vi "定点周期设置.vi"(11 "TimingControl 输入":refnum<class "TimingControl.lvclass">) -> (3 "TimingControl 输出":refnum<class "TimingControl.lvclass">)   [LabVIEW 2016, in "ZKTimingControl.lvlib" / "TimingControl.lvclass"]
uses:
  TimingControl.lvclass
  <vilib>/Utility/miscctls.llb/LVPointTypeDef.ctl
  TimingControl.lvclass/TimingControl.ctl
  <vilib>/Utility/miscctls.llb/LVPositionTypeDef.ctl
panel:
  out "时间标识":timestamp format="%<%x %X>T"
  in  "每月启动":T1
  in  "每周启动":T2
  out "测试状态.结束时间":timestamp caption="结束时间" format="%<%y/%m/%d %H:%M:%S>T"
  out "测试状态.启动次数":dbl caption="启动次数"
  out "测试状态.启动时间":timestamp caption="启动时间" format="%<%y/%m/%d %H:%M:%S>T"
  in  "测量参数":T3={"氨氮"=TRUE, "总磷"=TRUE, "总氮"=TRUE, "CODMn"=TRUE, "CODCr"=FALSE, "氟化物"=FALSE, "挥发酚"=FALSE}
  in  "保存":bool
  in  "退出":bool
  in  "批量设置":bool
  out "周期模式选择卡":enum32{"选项卡 1", "选项卡 2"}(tab)
  in  "定点周期":T4
  in  "间隔启动":T6
  in  "周期模式":T7
  # "分钟"
  # "次"
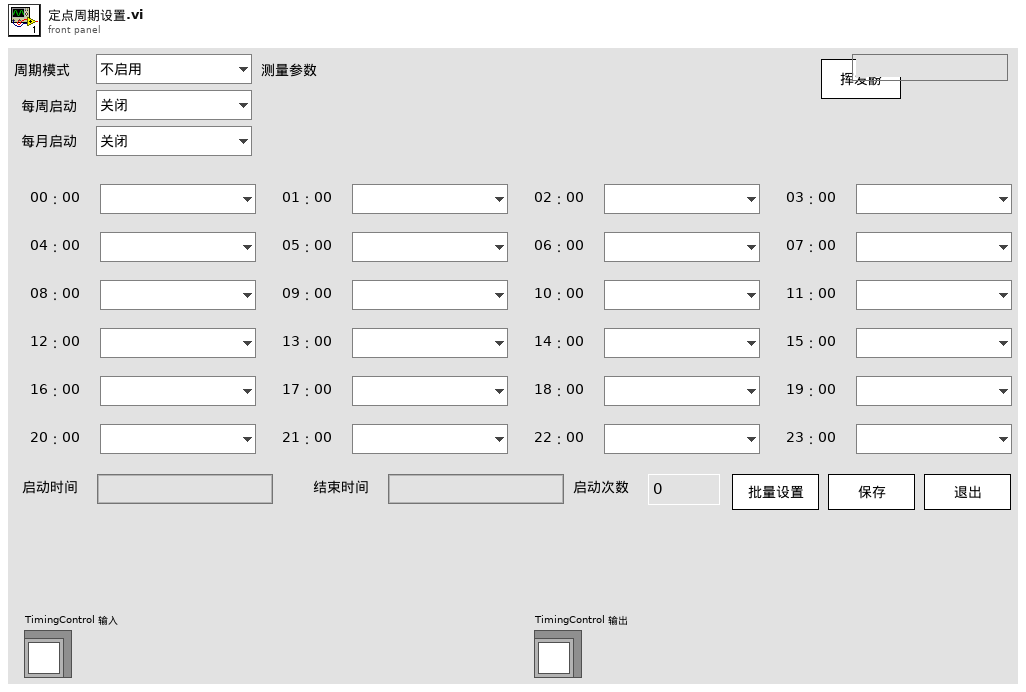
[diagram p1: front panel]
types:
  T1 = typedef "ZKTimingControl.lvlib/TimingControl.lvclass/每月启动.ctl" = enum16{"关闭", "1号", "2号", "3号", "4号", "5号", "6号", "7号", "8号", "9号", "10号", "11号", "12号", "13号", "14号", "15号", "16号", "17号", "18号", "19号", "20号", "21号", "22号", "23号", "24号", "25号", "26号", "27号", "28号", "29号", "30号", "31号"}
  T2 = typedef "ZKTimingControl.lvlib/TimingControl.lvclass/每周启动.ctl" = enum16{"关闭", "周日", "周一", "周二", "周三", "周四", "周五", "周六"}
  T3 = typedef "ZKTimingControl.lvlib/TimingControl.lvclass/测量参数.ctl" = cluster{"氨氮":bool, "总磷":bool, "总氮":bool, "CODMn":bool, "CODCr":bool, "氟化物":bool, "挥发酚":bool}
  T4 = typedef "ZKTimingControl.lvlib/TimingControl.lvclass/定点周期设置.ctl" = cluster{"启动命令":T5, "启动命令 2":T5, "启动命令 3":T5, "启动命令 4":T5, "启动命令 5":T5, "启动命令 6":T5, "启动命令 7":T5, "启动命令 8":T5, "启动命令 9":T5, "启动命令 10":T5, "启动命令 11":T5, "启动命令 12":T5, "启动命令 13":T5, "启动命令 14":T5, "启动命令 15":T5, "启动命令 16":T5, "启动命令 17":T5, "启动命令 18":T5, "启动命令 19":T5, "启动命令 20":T5, "启动命令 21":T5, "启动命令 22":T5, "启动命令 23":T5, "启动命令 24":T5}
  T5 = typedef "ZKTimingControl.lvlib/TimingControl.lvclass/启动命令选择.ctl" = enum16{"", "加标回收（启动采配水）", "加标回收（不启动采配水）", "水样测试（启动采配水）", "水样测试（不启动采配水）", "平行样测试（启动采配水）", "平行样测试（不启动采配水）", "集成干预测试"}
  T6 = typedef "ZKTimingControl.lvlib/TimingControl.lvclass/间隔启动设置.ctl" = cluster{"启动命令":T5, "启动间隔":dbl, "启动次数":i32}
  T7 = typedef "ZKTimingControl.lvlib/TimingControl.lvclass/周期模式设置.ctl" = enum16{"不启用", "定点模式", "间隔模式"}
  T8 = typedef "LVPointTypeDef.ctl" = cluster{"Horizontal":i16, "Vertical":i16}
  T9 = typedef "LVPositionTypeDef.ctl" = cluster{"Left":i32, "Top":i32}
  T10 = cluster{"启动时间":timestamp, "结束时间":timestamp, "启动次数":dbl}
  T11 = typedef "ZKTimingControl.lvlib/TimingControl.lvclass/State Data.ctl" = cluster{"仪器时间":timestamp, "仪器运行状态":bool, "配置文件路径":path, "测量参数":T3, "测试状态":cluster{"启动时间":timestamp, "结束时间":timestamp, "启动次数":dbl}, "配置信息":T12}
  T12 = typedef "ZKTimingControl.lvlib/TimingControl.lvclass/配置信息.ctl" = cluster{"每周启动":T2, "每月启动":T1, "周期模式":T7, "测量参数":T3, "定点周期":T4, "间隔启动":T6, "配置时间":timestamp}
  T13 = typedef "周期设置.lvlib/周期模式设置.ctl" = enum16{"不启用", "定点模式", "间隔模式"}
  T14 = cluster{"每周启动":T2, "每月启动":T1, "周期模式":T7, "测量参数":T3, "定点周期":T4, cluster{"启动命令":T5, "启动间隔":dbl, "启动次数":i32}, "seconds since 1Jan1904":timestamp}
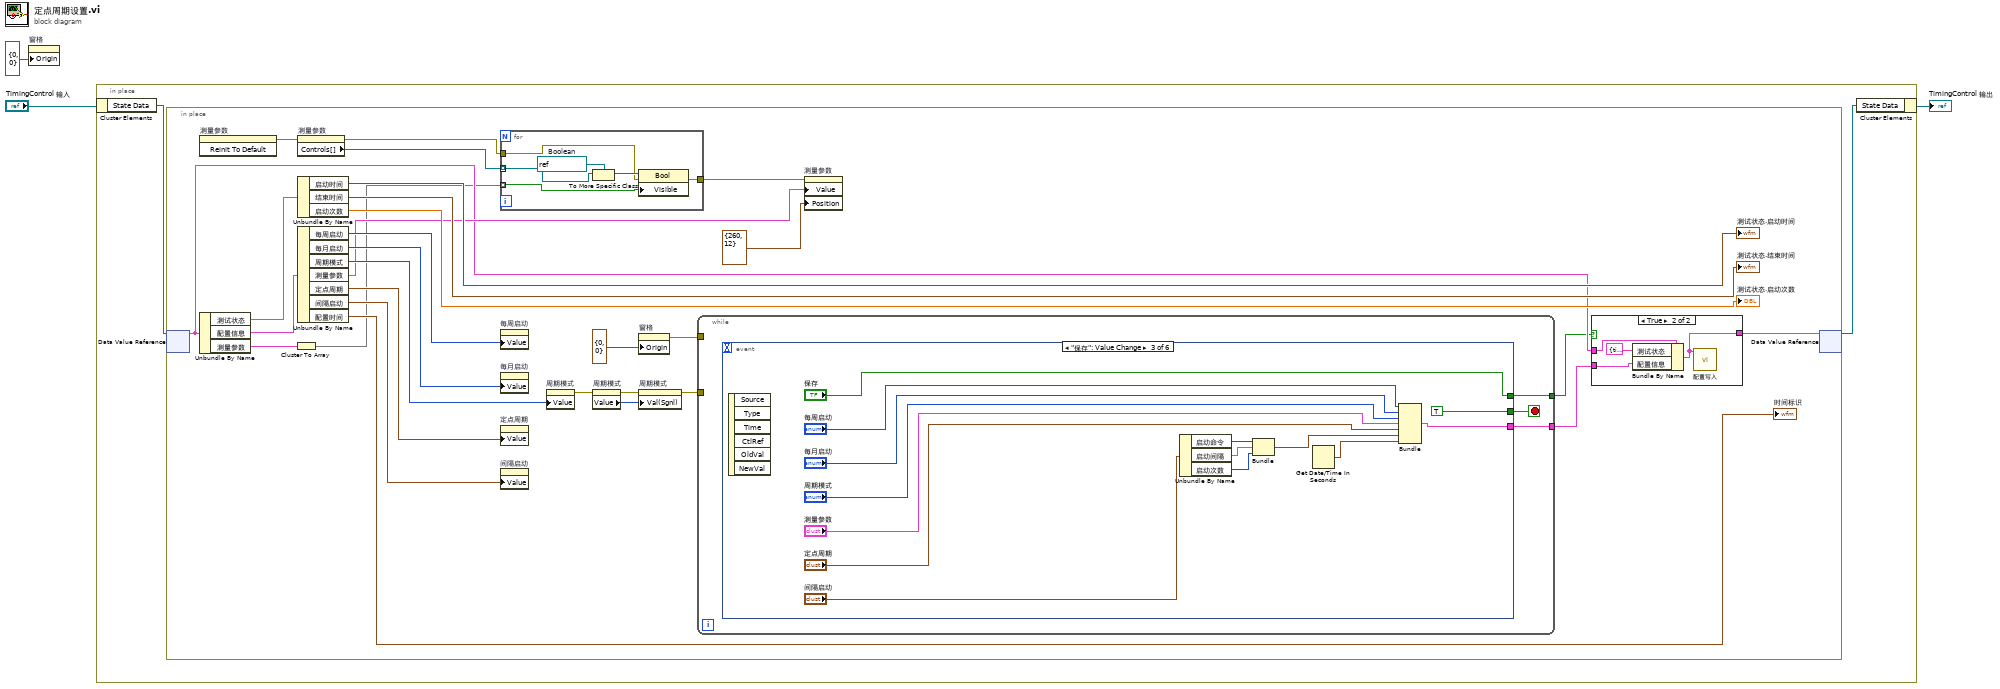
[diagram p0: block diagram]
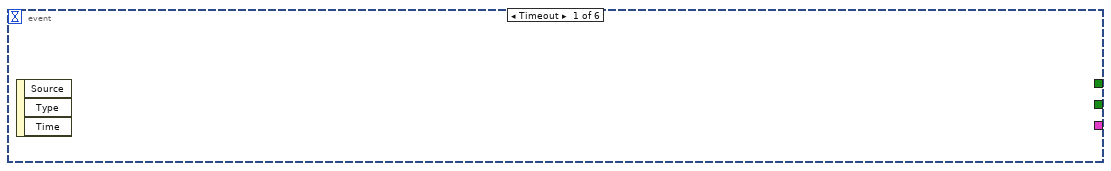
[diagram p3: hidden frame]
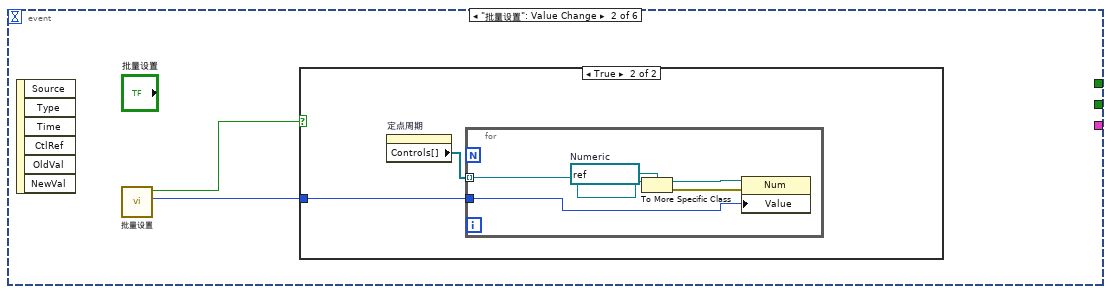
[diagram p4: hidden frame]
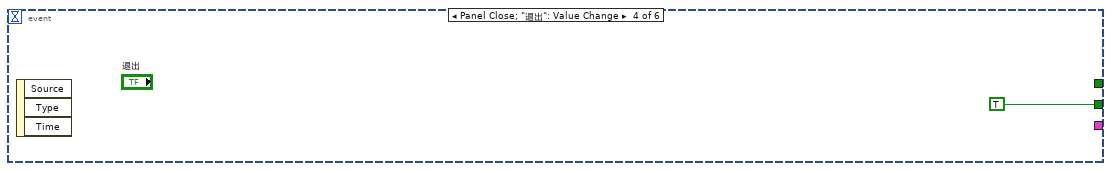
[diagram p6: hidden frame]
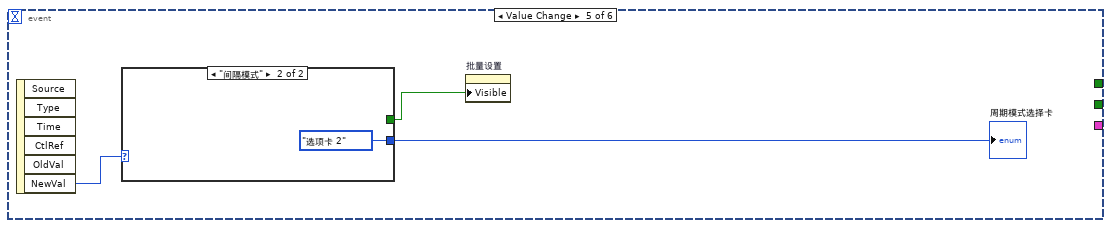
[diagram p7: hidden frame]
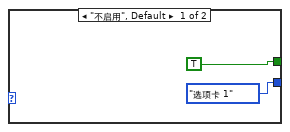
[diagram p8: hidden frame]
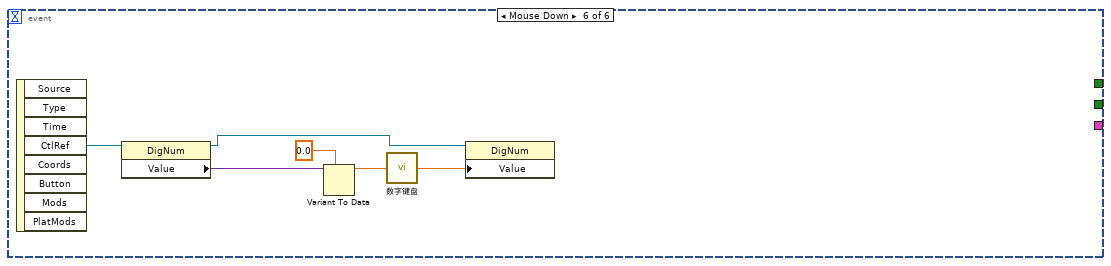
[diagram p9: hidden frame]
diagram:
  n1 = property on="窗格" class="Pane"("Origin"=T8 {"Horizontal"=0, "Vertical"=0} ("原点")) -> ()  [unwired: 2 in, 2 out]
  n2 = in-place {
    n3 = in-place-cluster #1("TimingControl 输入") -> ("State Data"=w5:refnum<data-value>)
    n4 = in-place {
      n5 = in-place-dvr #2(w5) -> (w17:T11)  [unwired: 1 out]
      n6 = invoke on="测量参数" class="Clust (strict)" method="Reinit To Default"() -> (error out=w9:errorcluster)  [unwired: 3 in, 2 out]
      n7 = Unbundle By Name(w17) -> ("测试状态"=w18:T10, "配置信息"=w19:T12, "测量参数"=w12:T3)
      n8 = Cluster To Array(cluster=w12) -> (array=w10:bool[])
      n9 = property on="测量参数" class="Clust (strict)"(error in=w9) -> (error out=w8:errorcluster, "Controls[]"=w11:refnum<vi>[])  [unwired: 1 in, 1 out]
      n10 = Unbundle By Name(w18) -> ("启动时间"=→"测试状态.启动时间":timestamp, "结束时间"=→"测试状态.结束时间":timestamp, "启动次数"=→"测试状态.启动次数":dbl)
      n11 = Unbundle By Name(w19) -> ("每周启动"=w25:T2, "每月启动"=w24:T1, "周期模式"=w26:T7, "测量参数"=w23:T3, "定点周期"=w22:T4, "间隔启动"=w21:T6, "配置时间"=→"时间标识":timestamp)
      n12 = for {
        tunnel: w11 -> [w40] mode=indexing
        tunnel: w10 -> [w39] mode=indexing
        tunnel: w8 -> [w36]
        tunnel: [w35] -> w7
        w37 = refnum<vi> refnum  # Boolean
        n13 = To More Specific Class(target class=w37, reference=w40) -> (specific class reference=w38:refnum<vi>)  [unwired: 1 in, 1 out]
        n14 = property class="Bool"(reference=w38, error in=w36, "Visible"=w39) -> (error out=w35:errorcluster)  [unwired: 1 out]
      }
      n15 = property on="每周启动" class="Enum (strict)"("Value"=w25) -> ()  [unwired: 2 in, 2 out]
      n16 = property on="每月启动" class="Enum (strict)"("Value"=w24) -> ()  [unwired: 2 in, 2 out]
      n17 = property on="定点周期" class="Clust (strict)"("Value"=w22) -> ()  [unwired: 2 in, 2 out]
      n18 = property on="间隔启动" class="Clust (strict)"("Value"=w21) -> ()  [unwired: 2 in, 2 out]
      n19 = property on="周期模式" class="Enum (strict)"("Value"=w26) -> (error out=w20:errorcluster)  [unwired: 2 in, 1 out]
      n20 = property on="周期模式" class="Enum (strict)"(error in=w20) -> (error out=w33:errorcluster, "Value"=w34:T13)  [unwired: 1 in, 1 out]
      n21 = property on="窗格" class="Pane"("Origin"=T8 {"Horizontal"=0, "Vertical"=0} ("原点")) -> (error out=w27:errorcluster)  [unwired: 2 in, 1 out]
      n22 = property on="周期模式" class="Enum (strict)"(error in=w33, "Val(Sgnl)"=w34) -> (error out=w32:errorcluster)  [unwired: 1 in, 1 out]
      n23 = while {
        tunnel: [w47] -> w15
        tunnel: w32 -> [_]
        tunnel: [w46] -> w14
        tunnel: w27 -> [_]
        stop <- w48 stop-if-true
        n24 = event shown="[2] \"保存\": Value Change" {
          selector: _ -> [_ _ _ _ _ _]
          dyn-events: _ -> [_ _ _ _ _ _]
          timeout: _ -> [_ _ _ _ _ _]
          tunnel: [_ _ TRUE TRUE _ _] -> w48
          tunnel: [_ _ w70 _ _ _] -> w47
          tunnel: [_ _ "保存" _ _ _] -> w46
          event Timeout {
            n25 = event-data() -> ()  [unwired: 1 in, 3 out]
          }
          event "批量设置": Value Change {
            n26 = event-data() -> ()  [unwired: 1 in, 6 out]
            n27 = call "批量设置.vi"() -> ("启动命令 2"=w50:T5, "确定 2"=w49:bool)  [unwired: 10 in]
            n28 = case shown="True" w49 {
              tunnel: w50 -> [_ w51]
              frame False {
              }
              frame True {
                n29 = property on="定点周期" class="Clust (strict)"() -> ("Controls[]"=w52:refnum<vi>[])  [unwired: 2 in, 2 out]
                n30 = for {
                  tunnel: w52 -> [w57] mode=indexing
                  tunnel: w51 -> [w53]
                  w56 = refnum<vi> refnum  # Numeric
                  n31 = To More Specific Class(target class=w56, reference=w57) -> (specific class reference=w55:refnum<vi>, error out=w54:errorcluster)  [unwired: 1 in]
                  n32 = property class="Num"(reference=w55, error in=w54, "Value"=w53) -> ()  [unwired: 2 out]
                }
              }
            }
          }
          event "保存": Value Change {
            n33 = event-data() -> ()  [unwired: 1 in, 6 out]
            n34 = Unbundle By Name("间隔启动") -> ("启动命令"=w67:T5, "启动间隔"=w66:dbl, "启动次数"=w65:i32)
            n35 = Bundle("启动命令"=w67, "启动间隔"=w66, "启动次数"=w65) -> (w64:cluster{"启动命令":T5, "启动间隔":dbl, "启动次数":i32})  [unwired: 1 in]
            n36 = Get Date/Time In Seconds() -> (seconds since 1Jan1904=w58:timestamp)
            n37 = Bundle("每周启动"="每周启动", "每月启动"="每月启动", "周期模式"="周期模式", "测量参数"="测量参数", "定点周期"="定点周期", w64, "seconds since 1Jan1904"=w58) -> (w70:T14)  [unwired: 1 in]
          }
          event Panel Close; "退出": Value Change {
            n38 = event-data() -> ()  [unwired: 1 in, 3 out]
          }
          event Value Change {
            n39 = event-data() -> ("NewVal"=w74:T7)  [unwired: 1 in, 5 out]
            n40 = case shown="\"间隔模式\"" w74 {
              tunnel: [TRUE ("可见") _] -> w75
              tunnel: [enum32{"选项卡 1", "选项卡 2"}."选项卡 1" ("周期模式选择卡") enum32{"选项卡 1", "选项卡 2"}."选项卡 2" ("周期模式选择卡")] -> w73
              frame "不启用", Default {
              }
              frame "间隔模式" {
              }
            }
            "周期模式选择卡" <- w73
            n41 = property on="批量设置" class="Bool"("Visible"=w75) -> ()  [unwired: 2 in, 2 out]
          }
          event Mouse Down {
            n42 = event-data() -> ("CtlRef"=w84:refnum<vi>)  [unwired: 1 in, 7 out]
            n43 = property class="DigNum"(reference=w84) -> (reference out=w83:refnum<vi>, "Value"=w82:variant)  [unwired: 1 in, 1 out]
            n44 = Variant To Data(type=0.0, Variant=w82) -> (data=w80:dbl)  [unwired: 1 in, 1 out]
            n45 = call "数字键盘.vi"("OldNumber"=w80) -> ("NewNumber"=w79:sgl)
            n46 = property class="DigNum"(reference=w83, "Value"=w79) -> ()  [unwired: 1 in, 2 out]
          }
        }
      }
      n47 = property on="测量参数" class="Clust (strict)"(error in=w7, "Value"=w23, "Position"=T9 {"Left"=260, "Top"=12} ("位置")) -> ()  [unwired: 1 in, 2 out]
      n48 = case shown="True" w14 {
        tunnel: w17 -> [w41 w45]
        tunnel: [w41 w42] -> w16
        tunnel: w15 -> [_ w44]
        frame False {
        }
        frame True {
          n49 = Bundle By Name(cluster=w45, "测试状态"=T10 {"启动时间"=timestamp(0 s since 1904-01-01), "结束时间"=timestamp(0 s since 1904-01-01), "启动次数"=0.0}, "配置信息"=w44) -> (w42:T11)
          n50 = call "配置写入.vi"("数据值"=w42) -> ()  [unwired: 10 in, 1 out]
        }
      }
      n51 = in-place-dvr #2(w16) -> (w4:refnum<data-value>)  [unwired: 1 out]
    }
    n52 = in-place-cluster #1("State Data"=w4) -> (→"TimingControl 输出":refnum<class "TimingControl.lvclass">)
  }
